vi "Generate Comments.vi"(7 "error in (no error)":errorcluster, 9 "reset comments":bool, 10 "Control Experiment":refnum<class "Control Experiment.lvclass">) -> (0 "error out":errorcluster, 2 "Comments":string, 3 "Control Experiment out":refnum<class "Control Experiment.lvclass">)   [LabVIEW 2019, in "Control Experiment.lvclass"]
uses:
  Control Experiment.lvclass
  Control Experiment.lvclass/Control Experiment.ctl
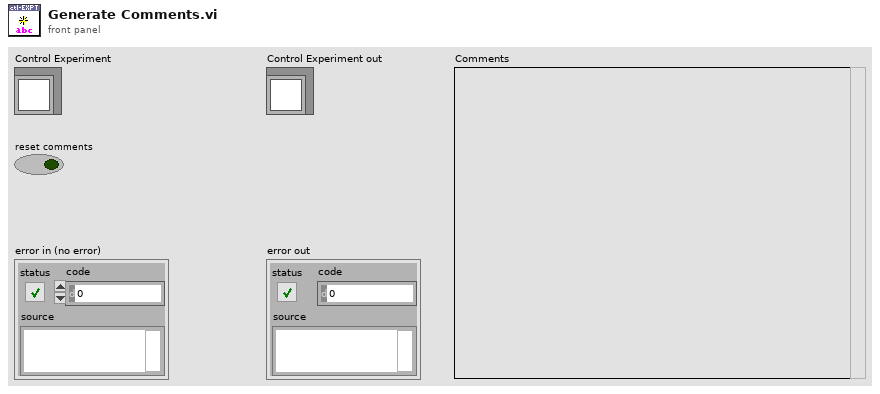
[diagram p1: front panel]
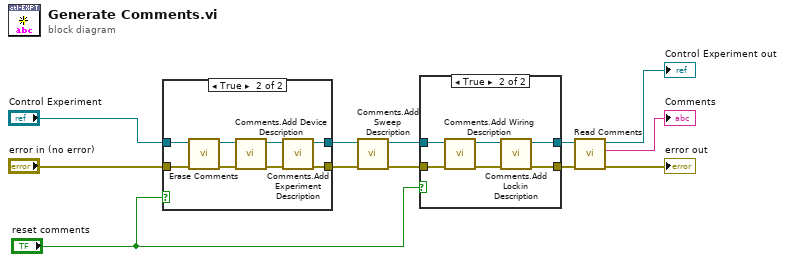
[diagram p0: block diagram]
diagram:
  n1 = case shown="True" "reset comments" {
    tunnel: "Control Experiment" -> [w14 w22]
    tunnel: "error in (no error)" -> [w13 w20]
    tunnel: [w14 w16] -> w11
    tunnel: [w13 w15] -> w10
    frame False {
    }
    frame True {
      n2 = call "Erase Comments.vi"("error in (no error)"=w20, "Control Experiment in"=w22) -> ("error out"=w19:errorcluster, "Control Experiment out"=w21:refnum<class "Control Experiment.lvclass">)  [unwired: 8 in]
      n3 = call "Comments.Add Device Description.vi"("error in (no error)"=w19, "Control Experiment in"=w21) -> ("error out"=w17:errorcluster, "Control Experiment out"=w18:refnum<class "Control Experiment.lvclass">)  [unwired: 8 in]
      n4 = call "Comments.Add Experiment Description.vi"("error in (no error)"=w17, "Control Experiment"=w18) -> ("error out"=w15:errorcluster, "Control Experiment out"=w16:refnum<class "Control Experiment.lvclass">)  [unwired: 7 in]
    }
  }
  n5 = call "Comments.Add Sweep Description.vi"("error in (no error)"=w10, "Control Experiment in"=w11) -> ("error out"=w8:errorcluster, "Control Experiment out"=w9:refnum<class "Control Experiment.lvclass">)  [unwired: 7 in, 1 out]
  n6 = case shown="True" "reset comments" {
    tunnel: w9 -> [w23 w28]
    tunnel: w8 -> [w24 w27]
    tunnel: [w24 w26] -> w7
    tunnel: [w23 w25] -> w6
    frame False {
    }
    frame True {
      n7 = call "Comments.Add Wiring Description.vi"("error in (no error)"=w27, "Control Experiment in"=w28) -> ("error out"=w29:errorcluster, "Control Experiment out"=w30:refnum<class "Control Experiment.lvclass">)  [unwired: 7 in, 1 out]
      n8 = call "Comments.Add Lockin Description.vi"("error in (no error)"=w29, "Control Experiment"=w30) -> ("error out"=w26:errorcluster, "Control Experiment out"=w25:refnum<class "Control Experiment.lvclass">)  [unwired: 7 in]
    }
  }
  n9 = call "Read Comments.vi"("error in (no error)"=w7, "Control Experiment in"=w6) -> ("error out"=→"error out":errorcluster, "Comments"=→"Comments":string, "Control Experiment out"=→"Control Experiment out":refnum<class "Control Experiment.lvclass">)  [unwired: 7 in]
